vi "Design Challenge Larry.vi"() -> ()   [LabVIEW 2025]
panel:
  out "XY Graph":cluster{"X":dbl, "Y":dbl}[](graph)
  in  "stop":bool
  in  "Clear":bool
  in  "Run":bool
  out "Linear Drag Coeff.":dbl
  in  "Drag Coefficient":dbl(slide) scale=0.0..0.2
  in  "Initial Height (m)":dbl(slide) scale=0.0..20.0
  in  "Initial Speed\n(m/s)":dbl
  in  "Mass (kg)":dbl
  in  "Launch Angle":dbl(knob) scale=0.0..89.0
  out "Launch Angle (deg)":dbl
  out "Initial Height (m)":dbl
  # "ME 235: Design of Microprocessor Based Mechanical Systems"
  # "Lab 2 - Design Challenge (Larry)"
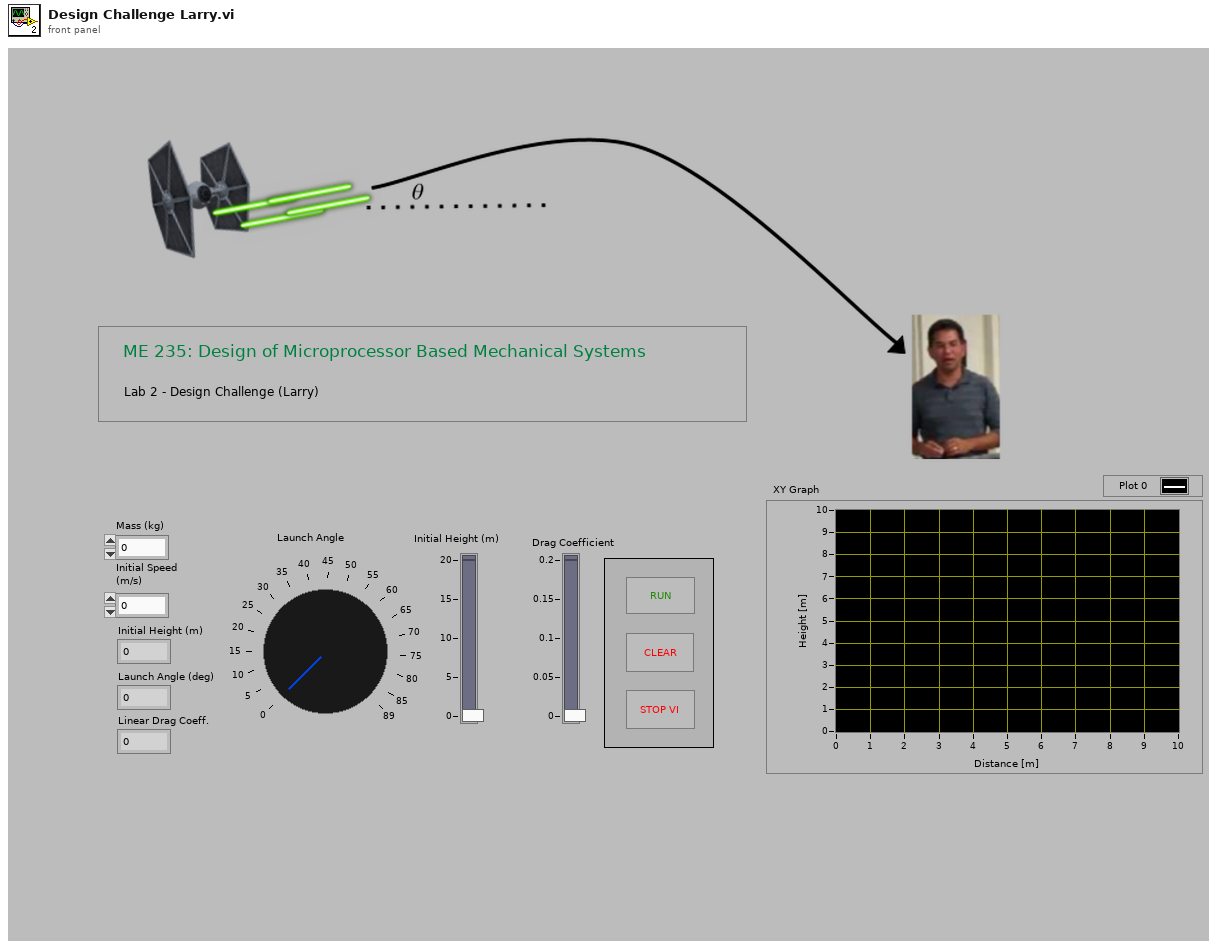
[diagram p1: front panel]
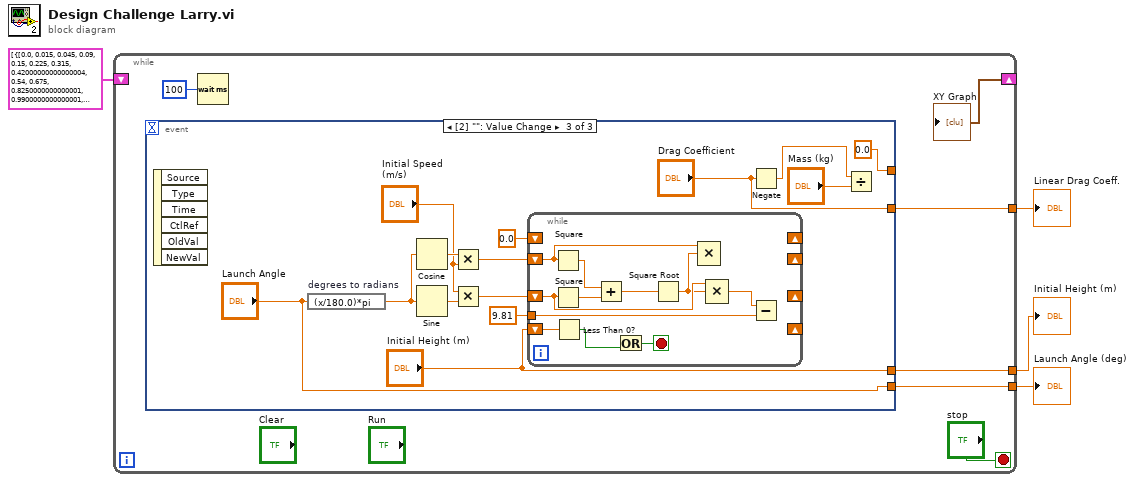
[diagram p0: block diagram]
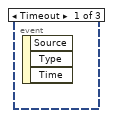
[diagram p2: hidden frame]
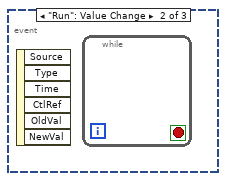
[diagram p3: hidden frame]
diagram:
  n1 = while {
    shift-right: ["XY Graph"] -> _
    shift-left: cluster{dbl[], dbl[]}[] [{[0.0, 0.015, 0.045, 0.09, 0.15, 0.225, 0.315, 0.42000000000000004, 0.54, 0.675, 0.8250000000000001, 0.9900000000000001, 1.1700000000000002, 1.3650000000000002, 1.5750000000000002, 1.8000000000000003, 2.04, 2.295, 2.565, 2.85, 3.1500000000000004, 3.4650000000000003, 3.7950000000000004, 4.140000000000001, 4.500000000000001, 4.875000000000001, 5.265000000000001, 5.670000000000001, 6.090000000000001, 6.525, 6.9750000000000005, 7.44, 7.92, 8.415, 8.924999999999999, 9.45, 9.989999999999998, 10.544999999999998, 11.114999999999998, 11.7, 12.299999999999999, 12.915, 13.545, 14.19, 14.85, 15.525, 16.215, 16.92, 17.64, 18.375, 19.125, 19.89, 20.67, 21.465000000000003, 22.275000000000002, 23.1, 23.94, 24.795, 25.665000000000003, 26.550000000000004, 27.450000000000003, 28.365000000000002, 29.295, 30.240000000000002, 31.200000000000003, 32.175000000000004, 33.165000000000006, 34.17000000000001, 35.19000000000001, 36.22500000000001, 37.275000000000006, 38.34, 39.42, 40.515, 41.625, 42.75, 43.89, 45.045, 46.215, 47.400000000000006, 48.60000000000001, 49.81500000000001, 51.04500000000001, 52.290000000000006, 53.550000000000004, 54.825, 56.115, 57.42, 58.74, 60.075, 61.425000000000004, 62.790000000000006, 64.17, 65.565, 66.975, 68.39999999999999, 69.83999999999999, 71.29499999999999, 72.76499999999999, 74.24999999999999, 75.74999999999999, 77.26499999999999, 78.79499999999999, 80.33999999999999, 81.89999999999999, 83.475, 85.065, 86.67, 88.29, 89.92500000000001, 91.57500000000002, 93.24000000000002, 94.92000000000003, 96.61500000000004, 98.32500000000003], [0.0, 6.02, 6.06, 6.1049999999999995, 6.164999999999999, 6.239999999999999, 6.329999999999999, 6.435, 6.555, 6.6899999999999995, 6.84, 7.005, 7.185, 7.38, 7.59, 7.8149999999999995, 8.055, 8.31, 8.58, 8.865, 9.165000000000001, 9.48, 9.81, 10.040000000000001, 10.280000000000001, 10.530000000000001, 10.790000000000001, 11.06, 11.34, 11.629999999999999, 11.93, 12.24, 12.56, 12.89, 13.23, 13.58, 13.94, 14.309999999999999, 14.69, 15.08, 15.48, 15.89, 16.310000000000002, 16.525000000000002, 16.745, 16.970000000000002, 17.200000000000003, 17.435000000000002, 17.675, 17.92, 18.17, 18.425, 18.685000000000002, 18.950000000000003, 19.220000000000002, 19.495, 19.775000000000002, 20.060000000000002, 20.35, 20.645000000000003, 20.945000000000004, 21.250000000000004, 21.560000000000002, 21.560000000000002, 21.560000000000002, 21.560000000000002, 21.560000000000002, 21.560000000000002, 21.560000000000002, 21.560000000000002, 21.560000000000002, 21.560000000000002, 21.560000000000002, 21.560000000000002, 21.560000000000002, 21.560000000000002, 21.560000000000002, 21.560000000000002, 21.560000000000002, 21.560000000000002, 21.560000000000002, 21.560000000000002, 21.560000000000002, 21.145000000000003, 20.725, 20.3, 19.87, 19.435000000000002, 18.995, 18.55, 18.1, 17.645000000000003, 17.185000000000002, 16.720000000000002, 16.250000000000004, 15.775000000000004, 15.295000000000003, 14.810000000000004, 14.320000000000004, 13.825000000000005, 13.325000000000005, 12.820000000000004, 12.310000000000004, 11.280000000000005, 10.240000000000006, 9.190000000000005, 8.130000000000004, 7.060000000000004, 5.980000000000004, 4.890000000000004, 3.7900000000000045, 2.6800000000000046, 1.5600000000000047, 0.4300000000000048, -0.7099999999999951]}, {[0.0, 0.025, 0.07500000000000001, 0.15000000000000002, 0.25, 0.375, 0.525, 0.7000000000000001, 0.9000000000000001, 1.125, 1.375, 1.65, 1.95, 2.275, 2.625, 3.0, 3.4, 3.825, 4.275, 4.75, 5.25, 5.775, 6.325, 6.9, 7.5, 8.125, 8.775, 9.450000000000001, 10.15, 10.875, 11.625, 12.4, 13.200000000000001, 14.025, 14.875, 15.75, 16.65, 17.575, 18.525, 19.5, 20.5, 21.525, 22.575, 23.65, 24.75, 25.875, 27.025, 28.2, 29.4, 30.625, 31.875, 33.15, 34.449999999999996, 35.775, 37.125, 38.5, 39.9, 41.324999999999996, 42.775, 44.25, 45.75, 47.275], [6.0, 6.005, 6.015, 6.029999999999999, 6.049999999999999, 6.074999999999999, 6.1049999999999995, 6.14, 6.18, 6.225, 6.2749999999999995, 6.329999999999999, 6.389999999999999, 6.454999999999999, 6.5249999999999995, 6.6, 6.68, 6.765, 6.765, 6.765, 6.765, 6.765, 6.765, 6.765, 6.765, 6.765, 6.765, 6.765, 6.765, 6.765, 6.765, 6.765, 6.765, 6.765, 6.765, 6.765, 6.765, 6.765, 6.574999999999999, 6.379999999999999, 6.179999999999999, 5.974999999999999, 5.764999999999999, 5.549999999999999, 5.329999999999999, 5.1049999999999995, 4.875, 4.64, 4.3999999999999995, 4.154999999999999, 3.9049999999999994, 3.6499999999999995, 3.3899999999999997, 3.1249999999999996, 2.8549999999999995, 2.5799999999999996, 2.3, 2.0149999999999997, 1.4349999999999998, 0.845, 0.2450000000000001, -0.36499999999999977]}] ("Trajectory Graph") -> [_]
    tunnel: [w7] -> w3
    tunnel: [w6] -> w2
    tunnel: [w5] -> w1
    stop <- "stop" stop-if-true
    n2 = event shown="[2] \"\": Value Change" {
      selector: _ -> [_ _ _]
      dyn-events: _ -> [_ _ _]
      timeout: _ -> [_ _ _]
      tunnel: [_ _ 0.0] -> _
      tunnel: [_ _ "Launch Angle"] -> w7
      tunnel: [_ _ "Initial Height (m)"] -> w6
      tunnel: [_ _ "Drag Coefficient"] -> w5
      event Timeout {
        n3 = event-data() -> ()  [unwired: 1 in, 3 out]
      }
      event "Run": Value Change {
        n4 = event-data() -> ()  [unwired: 1 in, 6 out]
        n5 = while {
          stop <- _ stop-if-true
        }
      }
      event "Clear": Value Change {
        n6 = event-data() -> ()  [unwired: 1 in, 6 out]
        n7 = expression code="(x/180.0)*pi" "degrees to radians"("Launch Angle") -> (w18:dbl)
        n8 = Cosine(x=w18) -> (cos(x)=w20:dbl)
        n9 = Sine(x=w18) -> (sin(x)=w19:dbl)
        n10 = Multiply(x=w20, y="Initial Speed\n(m/s)") -> (x*y=w23:dbl)
        n11 = Multiply(x="Initial Speed\n(m/s)", y=w19) -> (x*y=w22:dbl)
        n12 = while {
          shift-right: _ -> [_]
          shift-left: "Initial Height (m)" -> [w25]
          shift-right: _ -> [_]
          shift-left: 0.0 -> [_]
          shift-right: _ -> [_]
          shift-left: w23 -> [w32]
          shift-right: _ -> [_]
          shift-left: w22 -> [w31]
          tunnel: 9.81 -> [w28]
          stop <- w26 stop-if-true
          n13 = Square(x=w32) -> (x^2=w35:dbl)
          n14 = Square(x=w31) -> (x^2=w34:dbl)
          n15 = Less Than 0?(x=w25) -> (x < 0?=w27:bool)
          n16 = Add(x=w35, y=w34) -> (x+y=w33:dbl)
          n17 = Or(y=w27) -> (x .or. y?=w26:bool)  [unwired: 1 in]
          n18 = Square Root(x=w33) -> (sqrt(x)=w30:dbl)
          n19 = Compound Arithmetic op=MULTIPLY(w32, w30) -> ()  [unwired: 1 in, 1 out]
          n20 = Compound Arithmetic op=MULTIPLY(w31, w30) -> (w29:dbl)  [unwired: 1 in]
          n21 = Subtract(x=w29, y=w28) -> ()  [unwired: 1 out]
        }
        n22 = Negate(x="Drag Coefficient") -> (-x=w21:dbl)
        n23 = Divide(x=w21, y="Mass (kg)") -> ()  [unwired: 1 out]
      }
    }
    n24 = Wait (ms)(milliseconds to wait=u32 100) -> ()  [unwired: 1 out]
  }
  "Initial Height (m)" <- w2
  "Launch Angle (deg)" <- w3
  "Linear Drag Coeff." <- w1
